vi "CODcr测试流程.vi"(11 "输入参数":T1) -> ()   [LabVIEW 2016, in "CODCr库.lvlib"]
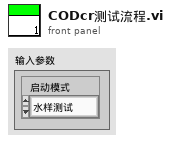
[diagram p1: front panel]
types:
  T1 = cluster{"启动模式":enum16{"水样测试", "空白核查", "跨度核查", "校零", "校标"}}
  T2 = enum16{"初始化", "通电", "测试启动", "等待测试完成", "测试完成", "断电", "结束"}
  T3 = cluster{"时间标识":timestamp, "设备":string, "日志信息":string, "流程参数":string}
  T4 = enum16{"空闲", "水样测试", "标样核查", "零点核查", "跨度核查", "空白测试", "平行样测试", "加标回收", "空白校准", "标样校准", "初始化（清洗）"}
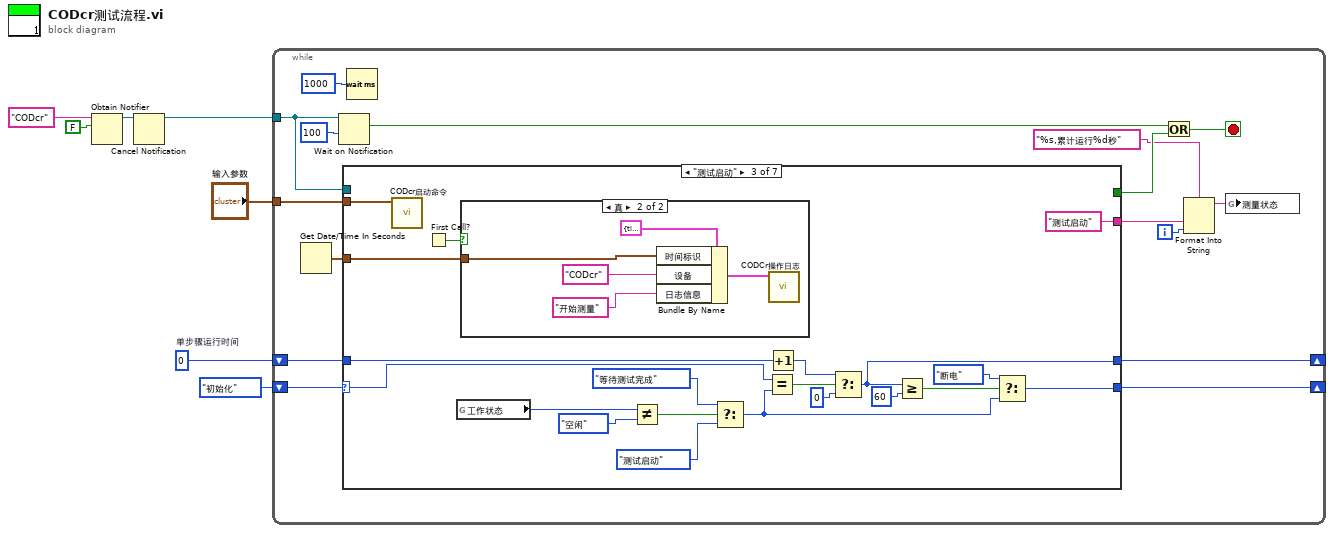
[diagram p0: block diagram]
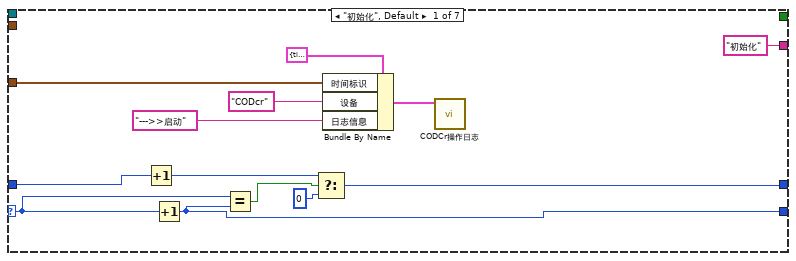
[diagram p2: hidden frame]
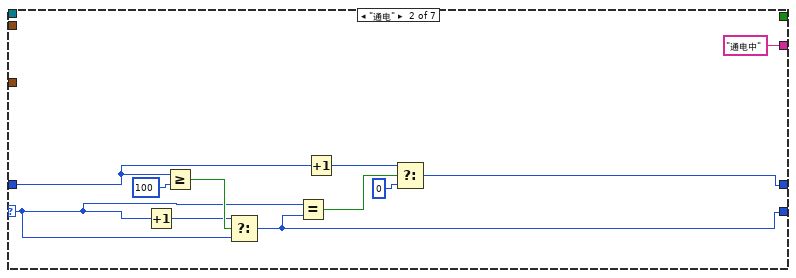
[diagram p3: hidden frame]
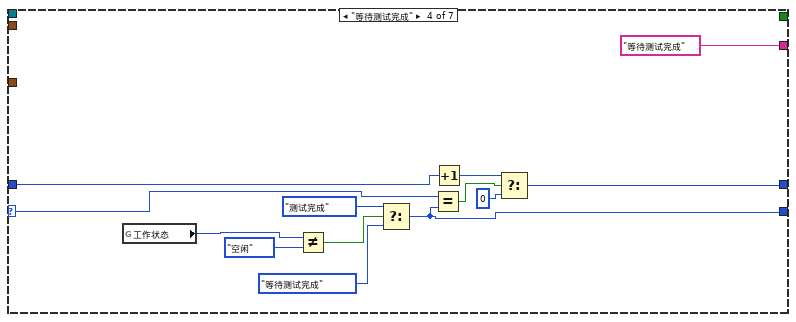
[diagram p5: hidden frame]
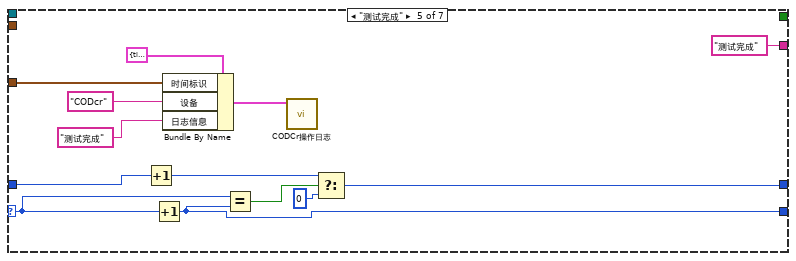
[diagram p6: hidden frame]
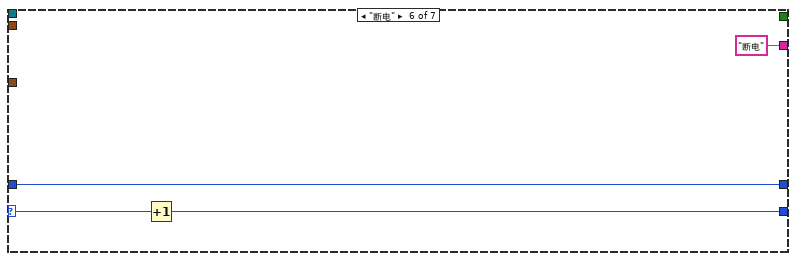
[diagram p7: hidden frame]
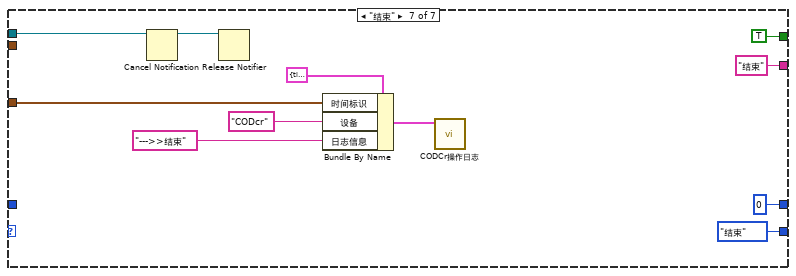
[diagram p8: hidden frame]
diagram:
  w6 = 0  # 单步骤运行时间
  n1 = Obtain Notifier(name (unnamed)="CODcr" ("名称（未命名）"), notification data type=FALSE) -> (notifier out=w3:refnum<notifier>)  [unwired: 2 in, 2 out]
  n2 = Cancel Notification(0:w3) -> (8:w2:refnum<notifier>)  [unwired: 1 in, 2 out]
  n3 = while {
    shift-right: [w22] -> _
    shift-left: T2."初始化" ("枚举") -> [w23]
    shift-right: [w20] -> _
    shift-left: w6 -> [w21]
    tunnel: w2 -> [w19]
    tunnel: "输入参数" -> [w14]
    i -> [w9]
    stop <- w15 stop-if-true
    n4 = Get Date/Time In Seconds() -> (seconds since 1Jan1904=w12:timestamp)
    n5 = Wait on Notification(notifier=w19, timeout in ms (-1)=100 ("超时毫秒(-1)")) -> (notification=w16:bool)  [unwired: 2 in, 3 out]
    n6 = case shown="\"测试启动\"" w23 {
      selector: w23 -> [w34 w41 w63 w80 w95 w101 _]
      tunnel: [_ _ _ _ _ _ TRUE] -> w17
      tunnel: [w35 w40 w52 w79 w94 w100 T2."结束" ("枚举")] -> w22
      tunnel: w21 -> [w36 w42 w64 w82 w96 w102 _]
      tunnel: [w32 w43 w57 w81 w97 w102 0 ("t")] -> w20
      tunnel: w19 -> [_ _ _ _ _ _ w110]
      tunnel: w14 -> [_ _ w51 _ _ _ _]
      tunnel: w12 -> [w28 _ w60 _ w88 _ w105]
      tunnel: ["初始化" ("测量状态") "通电中" ("测量状态") "测试启动" ("测量状态") "等待测试完成" ("测量状态") "测试完成" ("测量状态") "断电" ("测量状态") "结束" ("测量状态")] -> w10
      frame "初始化", Default {
        n7 = Increment(x=w36) -> (x+1=w30:i32)
        n8 = Increment(x=w34) -> (x+1=w35:T2)
        n9 = Equal?(x=w34, y=w35) -> (x = y?=w33:bool)
        n10 = Select(t=w30, s=w33, f=0 ("t")) -> (s? t:f=w32:i32)
        n11 = Bundle By Name(cluster=T3 {"时间标识"=timestamp(0 s since 1904-01-01), "设备"="", "日志信息"="", "流程参数"=""} ("data in"), "时间标识"=w28, "设备"="CODcr", "日志信息"="--->>启动") -> (w24:T3)
        n12 = call "CODCr操作日志.vi"("data in"=w24) -> ()  [unwired: 11 in]
      }
      frame "通电" {
        n13 = Increment(x=w41) -> (x+1=w45:T2)
        n14 = Greater Or Equal?(x=w42, y=100) -> (x >= y?=w46:bool)
        n15 = Select(t=w45, s=w46, f=w41) -> (s? t:f=w40:T2)
        n16 = Equal?(x=w41, y=w40) -> (x = y?=w44:bool)
        n17 = Increment(x=w42) -> (x+1=w39:i32)
        n18 = Select(t=w39, s=w44, f=0 ("t")) -> (s? t:f=w43:i32)
      }
      frame "测试启动" {
        n19 = call "CODcr启动命令.vi"("输入参数"=w51) -> ()  [unwired: 11 in]
        n20 = First Call?() -> (First Call?: T/F=w59:bool)
        n21 = global read "CODcr全局变量.vi" "工作状态"() -> (w50:T4)
        n22 = case shown="真" w59 {
          tunnel: w60 -> [_ w69]
          frame False {
          }
          frame True {
            n23 = Bundle By Name(cluster=T3 {"时间标识"=timestamp(0 s since 1904-01-01), "设备"="", "日志信息"="", "流程参数"=""} ("data in"), "时间标识"=w69, "设备"="CODcr", "日志信息"="开始测量") -> (w68:T3)
            n24 = call "CODCr操作日志.vi"("data in"=w68) -> ()  [unwired: 11 in]
          }
        }
        n25 = Not Equal?(x=w50, y=T4."空闲" ("工作状态")) -> (x != y?=w48:bool)
        n26 = Select(t=T2."等待测试完成" ("枚举"), s=w48, f=T2."测试启动" ("枚举")) -> (s? t:f=w54:T2)
        n27 = Equal?(x=w63, y=w54) -> (x = y?=w65:bool)
        n28 = Increment(x=w64) -> (x+1=w61:i32)
        n29 = Select(t=w61, s=w65, f=0 ("t")) -> (s? t:f=w57:i32)
        n30 = Greater Or Equal?(x=w57, y=60) -> (x >= y?=w55:bool)
        n31 = Select(t=T2."断电" ("枚举"), s=w55, f=w54) -> (s? t:f=w52:T2)
      }
      frame "等待测试完成" {
        n32 = global read "CODcr全局变量.vi" "工作状态"() -> (w75:T4)
        n33 = Not Equal?(x=w75, y=T4."空闲" ("工作状态")) -> (x != y?=w73:bool)
        n34 = Select(t=T2."测试完成" ("枚举"), s=w73, f=T2."等待测试完成" ("枚举")) -> (s? t:f=w79:T2)
        n35 = Equal?(x=w80, y=w79) -> (x = y?=w83:bool)
        n36 = Increment(x=w82) -> (x+1=w77:i32)
        n37 = Select(t=w77, s=w83, f=0 ("t")) -> (s? t:f=w81:i32)
      }
      frame "测试完成" {
        n38 = Increment(x=w96) -> (x+1=w92:i32)
        n39 = Increment(x=w95) -> (x+1=w94:T2)
        n40 = Bundle By Name(cluster=T3 {"时间标识"=timestamp(0 s since 1904-01-01), "设备"="", "日志信息"="", "流程参数"=""} ("data in"), "时间标识"=w88, "设备"="CODcr", "日志信息"="测试完成") -> (w86:T3)
        n41 = Equal?(x=w95, y=w94) -> (x = y?=w98:bool)
        n42 = call "CODCr操作日志.vi"("data in"=w86) -> ()  [unwired: 11 in]
        n43 = Select(t=w92, s=w98, f=0 ("t")) -> (s? t:f=w97:i32)
      }
      frame "断电" {
        n44 = Increment(x=w101) -> (x+1=w100:T2)
      }
      frame "结束" {
        n45 = Cancel Notification(0:w110) -> (8:w109:refnum<notifier>)  [unwired: 1 in, 2 out]
        n46 = Release Notifier(notifier=w109) -> ()  [unwired: 2 in, 3 out]
        n47 = Bundle By Name(cluster=T3 {"时间标识"=timestamp(0 s since 1904-01-01), "设备"="", "日志信息"="", "流程参数"=""} ("data in"), "时间标识"=w105, "设备"="CODcr", "日志信息"="--->>结束") -> (w103:T3)
        n48 = call "CODCr操作日志.vi"("data in"=w103) -> ()  [unwired: 11 in]
      }
    }
    n49 = Wait (ms)(milliseconds to wait=u32 1000 ("等待时间（毫秒）")) -> ()  [unwired: 1 out]
    n50 = Or(x=w16, y=w17) -> (x .or. y?=w15:bool)
    n51 = Format Into String(format string="%s,累计运行%d秒" ("格式字符串"), w10, w9) -> (resulting string=w8:string)  [unwired: 2 in, 1 out]
    n52 = global write "CODcr全局变量.vi" "测量状态"(w8) -> ()
  }
